vi "Library MCListBox Resizer.vi"(0 "MCListbox Refnum":refnum<vi>) -> ()   [LabVIEW 2012]
doc: "Changes the width of the active columns in a MCListBox relative to the width of all other resizeable columns. A column is resizeable when the 'Header String' of that column ends with a 'space' character. A column is active when it has a non-empty 'Header String'.\nSimply insert this VI as a sub VI and connect a 'MCListBox Refnum' to its front pane. Call this VI when the listbox has or might have resized."
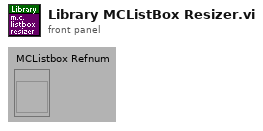
[diagram p1: front panel]
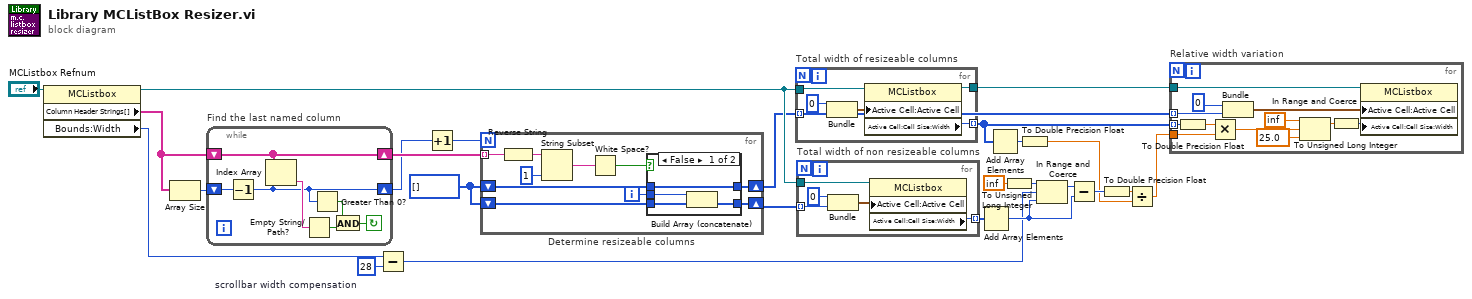
[diagram p0: block diagram]
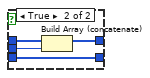
[diagram p2: hidden frame]
diagram:
  w21 = i32[] []
  w22 = u32 28  # scrollbar width compensation
  n1 = property class="MCListbox"(reference="MCListbox Refnum") -> (reference out=w24:refnum<vi>, "Column Header Strings[]"=w4:string[], "Bounds:Width"=w23:u32)  [unwired: 1 in, 1 out]
  n2 = Array Size(array=w4) -> (size(s)=w3:i32)
  n3 = while "Find the last named column" {
    shift-right: [w32] -> w5
    shift-left: w4 -> [w32]
    shift-right: [w28] -> w1
    shift-left: w3 -> [w31]
    stop <- w27 continue-if-true
    n4 = Decrement(x=w31) -> (x-1=w28:i32)
    n5 = Index Array(array=w32, index=w28) -> (element=w30:string)
    n6 = Empty String/Path?(string/path=w30) -> (empty?=w29:bool)
    n7 = Greater Than 0?(x=w28) -> (x > 0?=w26:bool)
    n8 = And(x=w26, y=w29) -> (x .and. y?=w27:bool)
  }
  n9 = Subtract(x=w23, y=w22) -> (x-y=w7:u32)
  n10 = Increment(x=w1) -> (x+1=w2:i32)
  n11 = for "Determine resizeable columns" {
    N: w2 -> [_]
    tunnel: w5 -> [w42] mode=indexing
    shift-right: [w39] -> w18
    shift-left: w21 -> [w38]
    shift-right: [w35] -> w20
    shift-left: w21 -> [w36]
    i -> [w37]
    n12 = Reverse String(1:w42) -> (0:w41:string)
    n13 = String Subset(string=w41, length (rest)=1 ("length (rest)")) -> (substring=w34:string)  [unwired: 1 in]
    n14 = White Space?(1:w34) -> (0:w33:bool)
    n15 = case shown="False" w33 {
      tunnel: [w46 w48] -> w39
      tunnel: w38 -> [w46 w50]
      tunnel: w37 -> [w45 w49]
      tunnel: w36 -> [w44 w47]
      tunnel: [w43 w47] -> w35
      frame False {
        n16 = Build Array (concatenate)(w45, w44) -> (w43:i32[])
      }
      frame True {
        n17 = Build Array (concatenate)(w50, w49) -> (w48:i32[])
      }
    }
  }
  n18 = for "Total width of resizeable columns" {
    tunnel: w24 -> [w54]
    tunnel: w18 -> [w53] mode=indexing
    tunnel: [w52] -> w17 mode=indexing
    tunnel: [w51] -> w19
    n19 = Bundle(0, w53) -> (w56:cluster{i32, i32})  [unwired: 1 in]
    n20 = property class="MCListbox"(reference=w54, "Active Cell:Active Cell"=w56) -> (reference out=w51:refnum<vi>, "Active Cell:Cell Size:Width"=w52:u32)  [unwired: 1 in, 1 out]
  }
  n21 = for "Total width of non resizeable columns" {
    tunnel: w24 -> [w61]
    tunnel: w20 -> [w59] mode=indexing
    tunnel: [w57] -> w14 mode=indexing
    n22 = Bundle(0, w59) -> (w60:cluster{i32, i32})  [unwired: 1 in]
    n23 = property class="MCListbox"(reference=w61, "Active Cell:Active Cell"=w60) -> ("Active Cell:Cell Size:Width"=w57:u32)  [unwired: 1 in, 2 out]
  }
  n24 = Add Array Elements(numeric array=w14) -> (sum=w10:u32)
  n25 = Add Array Elements(numeric array=w17) -> (sum=w13:u32)
  n26 = To Unsigned Long Integer(number=inf) -> (unsigned 32bit integer=w8:u32)
  n27 = To Double Precision Float(number=w13) -> (double precision float=w12:dbl)
  n28 = In Range and Coerce(upper limit=w8, x=w7, lower limit=w10) -> (coerced(x)=w6:u32)  [unwired: 1 out]
  n29 = Subtract(x=w6, y=w10) -> (x-y=w16:u32)
  n30 = To Double Precision Float(number=w16) -> (double precision float=w11:dbl)
  n31 = Divide(x=w11, y=w12) -> (x/y=w15:dbl)
  n32 = for "Relative width variation" {
    tunnel: w19 -> [w73]
    tunnel: w18 -> [w70] mode=indexing
    tunnel: w17 -> [w68] mode=indexing
    tunnel: w15 -> [w69]
    n33 = To Double Precision Float(number=w68) -> (double precision float=w67:dbl)
    n34 = Multiply(x=w67, y=w69) -> (x*y=w66:dbl)
    n35 = Bundle(0, w70) -> (w71:cluster{i32, i32})  [unwired: 1 in]
    n36 = In Range and Coerce(upper limit=inf, x=w66, lower limit=25.0) -> (coerced(x)=w65:dbl)  [unwired: 1 out]
    n37 = To Unsigned Long Integer(number=w65) -> (unsigned 32bit integer=w64:u32)
    n38 = property class="MCListbox"(reference=w73, "Active Cell:Active Cell"=w71, "Active Cell:Cell Size:Width"=w64) -> ()  [unwired: 1 in, 2 out]
  }
